vi "CreatePizza.vi"(8 "error in (no error)":errorcluster, 10 "PizzaId":T1, 11 "NYPizzaStore":refnum<class "NYPizzaStore.lvclass">) -> (0 "error out":errorcluster, 2 "Pizza":refnum<class "Pizza.lvclass">, 3 "NYPizzaStore":refnum<class "NYPizzaStore.lvclass">)   [LabVIEW 2020, in "FactoryMethod.lvlib" / "PizzaFactoryMethod.lvlib" / "NYPizzaStore.lvclass"]
uses:
  NYPizzaStore.lvclass
  Pizza/Pizza.lvclass
  PizzaStore/TypeDef/PizzaId.ctl
  NYStyleCheesePizza/NYStyleCheesePizza.lvclass
  E:/Francesco/GitHub/Design-Patterns-GoF_-_NI-LV/Creational/FactoryMethod/Head-First_Example/PizzaFactoryMethod/Pizza/Pizza.lvclass
  NYStyleClamPizza/NYStyleClamPizza.lvclass
  NYStylePepperoniPizza/NYStylePepperoniPizza.lvclass
  NYStyleVeggiePizza/NYStyleVeggiePizza.lvclass
  PizzaStore/PizzaStore.lvclass
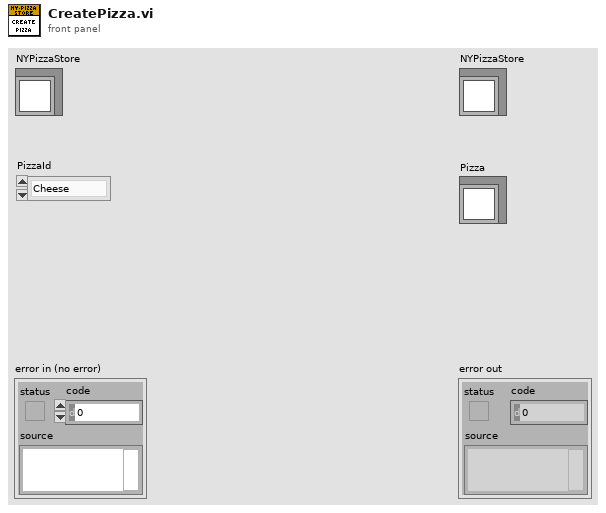
[diagram p1: front panel]
types:
  T1 = typedef "FactoryMethod.lvlib/PizzaFactoryMethod.lvlib/PizzaStore.lvclass/PizzaId.ctl" = enum16{"Cheese", "Clam", "Pepperoni", "Veggie"}
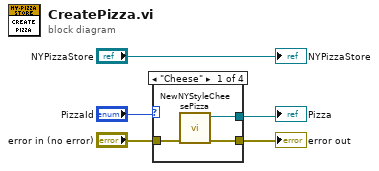
[diagram p0: block diagram]
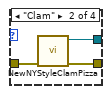
[diagram p2: hidden frame]
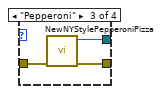
[diagram p3: hidden frame]
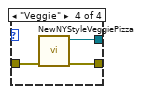
[diagram p4: hidden frame]
diagram:
  n1 = case shown="\"Cheese\"" "PizzaId" {
    tunnel: "error in (no error)" -> [w8 w11 w12 w15]
    tunnel: [w7 w10 w14 w17] -> w3
    tunnel: [w6 w9 w13 w16] -> w2
    frame "Cheese" {
      n2 = call "NewNYStyleCheesePizza.vi"("error in (no error)"=w8) -> ("error out"=w7:errorcluster, "NYStyleCheesePizza"=w6:refnum<class "NYStyleCheesePizza.lvclass">)  [unwired: 9 in]
    }
    frame "Clam" {
      n3 = call "NewNYStyleClamPizza.vi"("error in (no error)"=w11) -> ("error out"=w10:errorcluster, "NYStyleClamPizza"=w9:refnum<class "NYStyleClamPizza.lvclass">)  [unwired: 9 in]
    }
    frame "Pepperoni" {
      n4 = call "NewNYStylePepperoniPizza.vi"("error in (no error)"=w12) -> ("error out"=w14:errorcluster, "NYStylePepperoniPizza"=w13:refnum<class "NYStylePepperoniPizza.lvclass">)  [unwired: 9 in]
    }
    frame "Veggie" {
      n5 = call "NewNYStyleVeggiePizza.vi"("error in (no error)"=w15) -> ("error out"=w17:errorcluster, "NYStyleVeggiePizza"=w16:refnum<class "NYStyleVeggiePizza.lvclass">)  [unwired: 9 in]
    }
  }
  "error out" <- w3
  "Pizza" <- w2
  "NYPizzaStore" <- "NYPizzaStore"
